vi "CoomandPSOC.vi"(6 "ByteReceived":u32, 8 "error in (no error)":errorcluster, 9 "data":u8[](array[numeric]) format="%x", 10 "command":u8=5, 11 "VISA resource name":refnum<visa-resource-name>="COM7") -> (0 "error out":errorcluster, 2 "Command Echo":u8[](array[numeric]) format="%x", 3 "VISA resource name out":refnum<visa-resource-name>)   [LabVIEW 2019]
panel:
  out "return count":u32
  out "unsigned byte array":u8[](array[numeric]) format="%x"
  out "read buffer":string
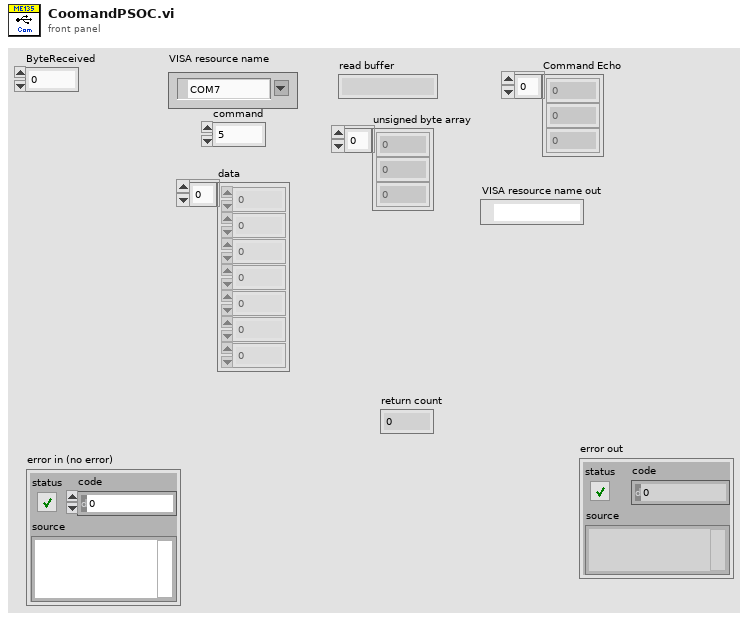
[diagram p1: front panel]
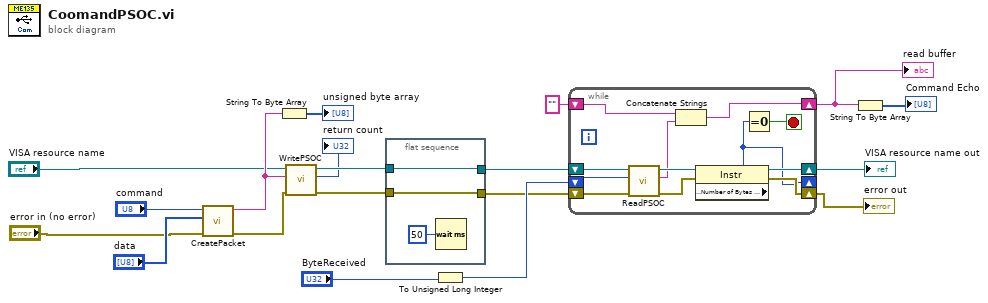
[diagram p0: block diagram]
diagram:
  n1 = call "CreatePacket.vi"("error in"="error in (no error)", "data"="data", "command"="command") -> ("error out"=w19:errorcluster, "Command String"=w10:string)  [unwired: 6 in, 1 out]
  n2 = String To Byte Array(string=w10) -> (unsigned byte array=→"unsigned byte array":u8[])
  n3 = call "WritePSOC.vi"("error in"=w19, "write buffer"=w10, "VISA resource name"="VISA resource name") -> ("error out"=w15:errorcluster, "return count"=→"return count":u32, "VISA resource name out"=w18:refnum<visa-resource-name>)  [unwired: 5 in]
  n4 = flat-sequence {
    tunnel: w18 -> [w22]
    tunnel: [w22] -> w17
    tunnel: [w20] -> w14
    tunnel: w15 -> [w20]
    frame #0 {
      n5 = Wait (ms)(milliseconds to wait=u32 50) -> ()  [unwired: 1 out]
    }
  }
  n6 = To Unsigned Long Integer(number="ByteReceived") -> (unsigned 32bit integer=w16:u32)
  n7 = while {
    shift-right: [w30] -> w7
    shift-left: w17 -> [w34]
    shift-right: [w28] -> w2
    shift-left: w14 -> [w32]
    shift-right: [w25] -> w6
    shift-left: "" -> [w24]
    shift-right: [w23] -> _
    shift-left: w16 -> [w33]
    stop <- w27 stop-if-true
    n8 = call "ReadPSOC.vi"("error in"=w32, "byte count"=w33, "VISA resource name"=w34) -> ("error out"=w29:errorcluster, "read buffer"=w26:string, "VISA resource name out"=w31:refnum<visa-resource-name>)  [unwired: 5 in]
    n9 = Concatenate Strings(w24, w26) -> (w25:string)
    n10 = property class="Instr"(reference=w31, error in=w29) -> (reference out=w30:refnum<visa-resource-name>, error out=w28:errorcluster, "Serial Settings:Number of Bytes at Serial Port"=w23:u32)
    n11 = Equal To 0?(x=w23) -> (x = 0?=w27:bool)
  }
  "read buffer" <- w6
  "error out" <- w2
  "VISA resource name out" <- w7
  n12 = String To Byte Array(string=w6) -> (unsigned byte array=→"Command Echo":u8[])
